vi "set sample rate.vi"(8 "error in (no error)":errorcluster, 10 "rate":u32, 11 "DevRefnum":u64) -> (0 "error out":errorcluster, 2 "real rate":u32, 3 "DevRefnum":u64)   [LabVIEW 2013, in "rtlsdr.lvlib"]
doc: "RTLSDR_API int rtlsdr_set_sample_rate(rtlsdr_dev_t *dev, uint32_t rate);"
uses:
  <instrlib>/rtlsdr/rtlsdr.lvlib
  <instrlib>/rtlsdr/VIs/rtlsdr.dll
panel:
  out "function return":i32
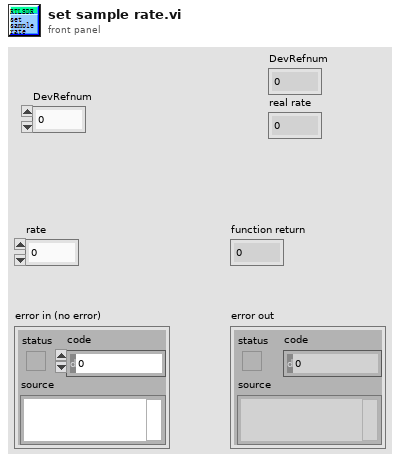
[diagram p1: front panel]
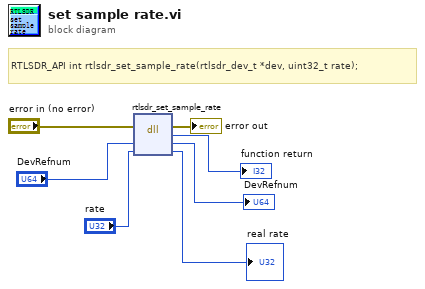
[diagram p0: block diagram]
diagram:
  # "RTLSDR_API int rtlsdr_set_sample_rate(rtlsdr_dev_t *dev, uint32_t rate);"
  n1 = dll-call lib="C:/Program Files (x86)/National Instruments/LabVIEW 2013/instr.lib/rtlsdr/VIs/rtlsdr.*" fn="rtlsdr_set_sample_rate"(error in="error in (no error)", "DevRefnum"="DevRefnum", "rate"="rate") -> (error out=→"error out":errorcluster, "return type"=→"function return":i32, "DevRefnum"=→"DevRefnum":u64, "rate"=→"real rate":u32)  [unwired: 2 in, 1 out]
